vi "Files Unopen and older then hours not in use check.vi"(9 "file extention list":string[](array[string]), 10 "Dir of Files to move and FTP":path, 11 "Time (Hours) last mod must be older then":dbl) -> (3 "Files to Archive and FTP":string[](array[string]))   [LabVIEW 2011]
doc: "Use this vi to deturmine a list of files in a directory that are have date modified dates older then the time you specify in hours, and that are currently not open by another application"
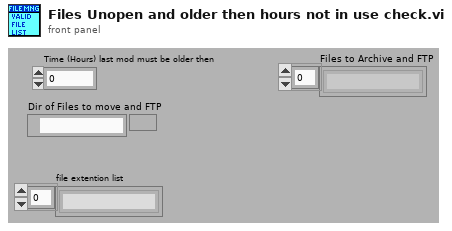
[diagram p1: front panel]
types:
  T1 = enum16{"open", "replace", "create", "open or create", "replace or create", "replace or create with confirmation"}
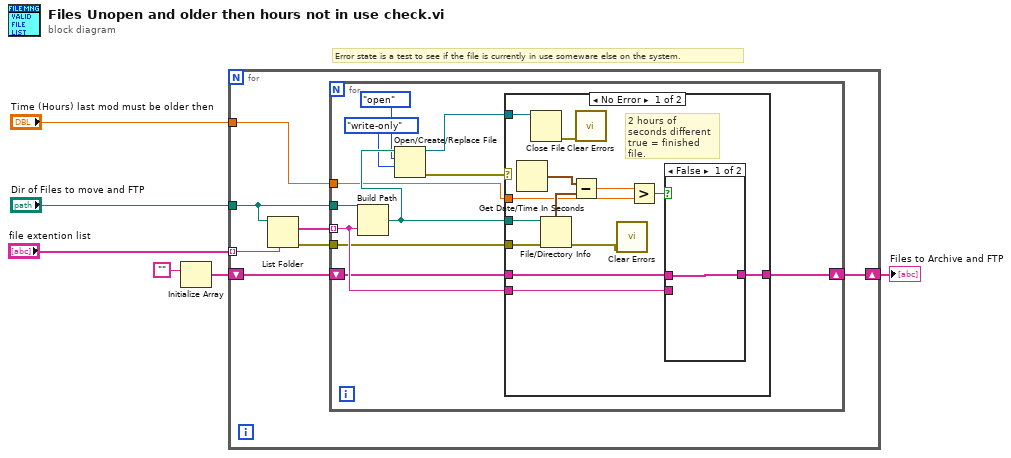
[diagram p0: block diagram]
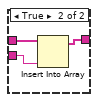
[diagram p2: hidden frame]
diagram:
  # "Error state is a test to see if the file is currently in use someware else on the system."
  n1 = Initialize Array("") -> (w3:string[])  [unwired: 1 in]
  n2 = for {
    tunnel: "Dir of Files to move and FTP" -> [w12]
    tunnel: "file extention list" -> [w11] mode=indexing
    tunnel: "Time (Hours) last mod must be older then" -> [w9]
    shift-right: [w7] -> w1
    shift-left: w3 -> [w8]
    n3 = List Folder(path=w12, pattern=w11) -> (filenames=w13:string[], error out=w10:errorcluster)  [unwired: 2 in, 2 out]
    n4 = for {
      tunnel: w13 -> [w23] mode=indexing
      tunnel: w12 -> [w24]
      tunnel: w10 -> [w22]
      tunnel: w9 -> [w16]
      shift-right: [w14] -> w7
      shift-left: w8 -> [w15]
      n5 = Build Path(base path=w24, name or relative path=w23) -> (appended path=w21:path)
      n6 = Open/Create/Replace File(file path (use dialog)=w21, operation (0:open)=T1."open", access (0:read/write)=enum16{"read/write", "read-only", "write-only"}."write-only") -> (refnum out=w17:refnum<file>, error out=w20:errorcluster)  [unwired: 3 in, 1 out]
      n7 = case shown="No Error" w20 {
        tunnel: w21 -> [w37 _]
        tunnel: w23 -> [w33 _]
        tunnel: w22 -> [w32 _]
        tunnel: w17 -> [w29 _]
        tunnel: w16 -> [w31 _]
        tunnel: w15 -> [w27 w42]
        tunnel: [w25 w42] -> w14
        frame No Error {
          # "2 hours of seconds different\ntrue = finished file."
          n8 = Get Date/Time In Seconds() -> (seconds since 1Jan1904=w36:timestamp)
          n9 = Close File(refnum=w29) -> (error out=w28:errorcluster)  [unwired: 1 in, 1 out]
          n10 = File/Directory Info(path=w37, error in=w32) -> (last mod=w35:timestamp, error out=w26:errorcluster)  [unwired: 5 out]
          n11 = Subtract(x=w36, y=w35) -> (x-y=w30:dbl)
          n12 = call <vilib>:"Clear Errors.vi"("error in (no error)"=w28) -> ()  [unwired: 6 in, 1 out]
          n13 = call <vilib>:"Clear Errors.vi"("error in (no error)"=w26) -> ()  [unwired: 6 in, 1 out]
          n14 = Greater?(x=w30, y=w31) -> (0:w34:bool)
          n15 = case shown="False" w34 {
            tunnel: w33 -> [_ w41]
            tunnel: w27 -> [w38 w40]
            tunnel: [w38 w39] -> w25
            frame False {
            }
            frame True {
              n16 = Insert Into Array(array=w40, new element=w41) -> (w39:string[])  [unwired: 1 in]
            }
          }
        }
        frame Error {
        }
      }
    }
  }
  "Files to Archive and FTP" <- w1
